vi "appendTable--double.vi"(8 "error in (no error)":errorcluster, 9 "Font":refnum<class "Style.lvclass">, 10 "Value":dbl[][](array[numeric]), 11 "MS-Excel in":refnum<class "MS-Excel.lvclass">) -> (0 "error out":errorcluster, 3 "MS-Excel out":refnum<class "MS-Excel.lvclass">)   [LabVIEW 2017, in "LabVIEW NPOI.lvlib" / "MS-Excel.lvclass"]
uses:
  MS-Excel.lvclass
  Styles/Style/Style.lvclass
  MS-Excel.lvclass/MS-Excel.ctl
  C:/Program Files (x86)/National Instruments/LabVIEW 2017/vi.lib/BenjaminR/LabVIEW NPOI/lib/NPOI 2.1.1/NPOI.dll
  Program Files (x86)/National Instruments/LabVIEW 2017/vi.lib/BenjaminR/LabVIEW NPOI/lib/NPOI 2.1.1/NPOI.dll
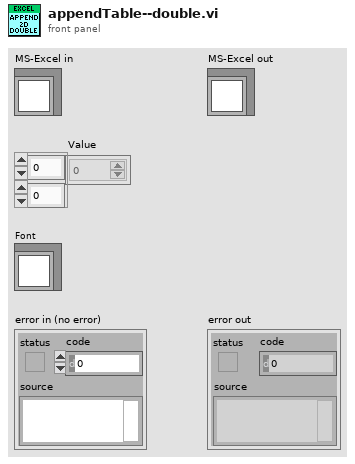
[diagram p1: front panel]
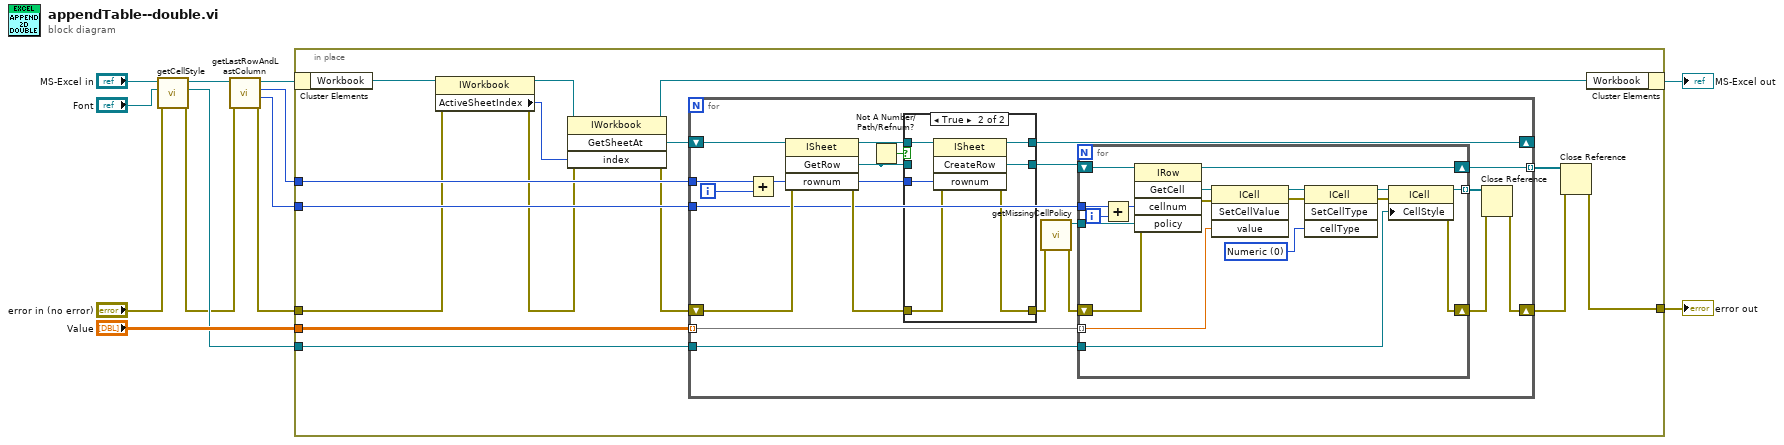
[diagram p0: block diagram]
diagram:
  n1 = call-dynamic "getCellStyle.vi"("error in (no error)"="error in (no error)", "Style"="Font", "MS-Excel in"="MS-Excel in") -> ("error out"=w1:errorcluster, "Cell Style"=w3:refnum<k24>, "MS-Excel out"=w5:refnum<class "MS-Excel.lvclass">)  [unwired: 6 in]
  n2 = call-dynamic "getLastRowAndLastColumn.vi"("error in (no error)"=w1, "MS-Excel in"=w5) -> ("error out"=w8:errorcluster, "Last Column"=w6:i32, "Last Row"=w7:i32, "MS-Excel out"=w9:refnum<class "MS-Excel.lvclass">)  [unwired: 6 in]
  n3 = in-place {
    in-place-border: w8 -> [w17]
    in-place-border: [w23] -> w12
    in-place-border: w7 -> [w28]
    in-place-border: w6 -> [w27]
    in-place-border: "Value" -> [w26]
    in-place-border: w3 -> [w14]
    n4 = in-place-cluster #1(w9) -> ("Workbook"=w15:refnum<k24>)
    n5 = property class="IWorkbook"(reference=w15, error in=w17) -> (reference out=w19:refnum<k24>, error out=w16:errorcluster, "ActiveSheetIndex"=w18:i32)
    n6 = invoke class="IWorkbook" method="GetSheetAt"(reference=w19, error in=w16, "index"=w18) -> (reference out=w21:refnum<k24>, error out=w20:errorcluster, "GetSheetAt"=w22:refnum<k24>)  [unwired: 1 in, 1 out]
    n7 = for {
      tunnel: w28 -> [w45]
      shift-right: [w44] -> _
      shift-left: w22 -> [w49]
      shift-right: [w35] -> w24
      shift-left: w20 -> [w42]
      tunnel: w27 -> [w39]
      tunnel: w26 -> [w38] mode=indexing
      tunnel: [w34] -> w25 mode=indexing
      tunnel: w14 -> [w29]
      i -> [w33]
      n8 = Add(x=w45, y=w33) -> (x+y=w40:i32)
      n9 = invoke class="ISheet" method="GetRow"(reference=w49, error in=w42, "rownum"=w40) -> (reference out=w46:refnum<k24>, error out=w43:errorcluster, "GetRow"=w47:refnum<k24>)  [unwired: 1 in, 1 out]
      n10 = Not A Number/Path/Refnum?(number/path/refnum=w47) -> (NaN/Path/Refnum?=w48:bool)
      n11 = case shown="True" w48 {
        tunnel: w47 -> [w69 _]
        tunnel: w46 -> [w68 w76]
        tunnel: w40 -> [_ w75]
        tunnel: w43 -> [w70 w71]
        tunnel: [w70 w73] -> w31
        tunnel: [w69 w74] -> w41
        tunnel: [w68 w72] -> w44
        frame False {
        }
        frame True {
          n12 = invoke class="ISheet" method="CreateRow"(reference=w76, error in=w71, "rownum"=w75) -> (reference out=w72:refnum<k24>, error out=w73:errorcluster, "CreateRow"=w74:refnum<k24>)  [unwired: 1 in, 1 out]
        }
      }
      n13 = call "getMissingCellPolicy.vi"("error in (no error)"=w31) -> ("error out"=w30:errorcluster, "CREATE_NULL_AS_BLANK"=w32:refnum<k24>)  [unwired: 9 in]
      n14 = for {
        shift-right: [w63] -> w34
        shift-left: w41 -> [w67]
        tunnel: w39 -> [w66]
        tunnel: w38 -> [w62] mode=indexing
        shift-right: [w50] -> w36
        shift-left: w30 -> [w61]
        tunnel: [w52] -> w37 mode=indexing
        tunnel: w32 -> [w55]
        tunnel: w29 -> [w53]
        i -> [w56]
        w57 = 0 items=["Numeric"=0, "String"=1, "Formula"=2, "Blank"=3, "Boolean"=4, "Error"=5, "Unknown"=-1] ("cellType")
        n15 = Add(x=w66, y=w56) -> (x+y=w65:i32)
        n16 = invoke class="IRow" method="GetCell"(reference=w67, error in=w61, "cellnum"=w65, "policy"=w55) -> (reference out=w63:refnum<k24>, error out=w60:errorcluster, "GetCell"=w64:refnum<k24>)  [unwired: 1 in, 2 out]
        n17 = invoke class="ICell" method="SetCellValue"(reference=w64, error in=w60, "value"=w62) -> (reference out=w59:refnum<k24>, error out=w58:errorcluster)  [unwired: 1 in, 2 out]
        n18 = invoke class="ICell" method="SetCellType"(reference=w59, error in=w58, "cellType"=w57) -> (reference out=w54:refnum<k24>, error out=w51:errorcluster)  [unwired: 1 in, 2 out]
        n19 = property class="ICell"(reference=w54, error in=w51, "CellStyle"=w53) -> (reference out=w52:refnum<k24>, error out=w50:errorcluster)
      }
      n20 = Close Reference(reference=w37, error in (no error)=w36) -> (error out=w35:errorcluster)
    }
    n21 = Close Reference(reference=w25, error in (no error)=w24) -> (error out=w23:errorcluster)
    n22 = in-place-cluster #1("Workbook"=w21) -> (→"MS-Excel out":refnum<class "MS-Excel.lvclass">)
  }
  "error out" <- w12
